vi "Options Changed.vi"(9 "error in (no error)":errorcluster, 13 "Setting ID":T1=enum."P 2") -> (8 "Settings Updated":bool, 10 "error out":errorcluster)   [LabVIEW 2011]
uses:
  Options PageID.ctl
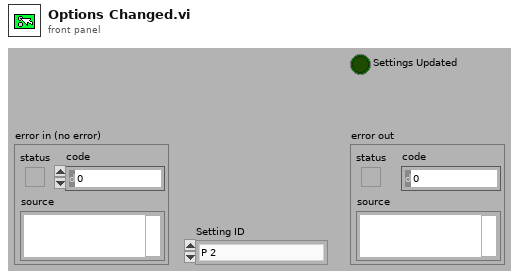
[diagram p1: front panel]
types:
  T1 = typedef "Options PageID.ctl" = enum16{"P 1 (App)", "P 2", "P 3", "P 4", "P 5", "P 6 (Err)", "P 7 (Expert)", "C 1", "C 2"}
  T2 = enum16{"Set Changed", "Changed?", "Init(numb in Prev..)"}
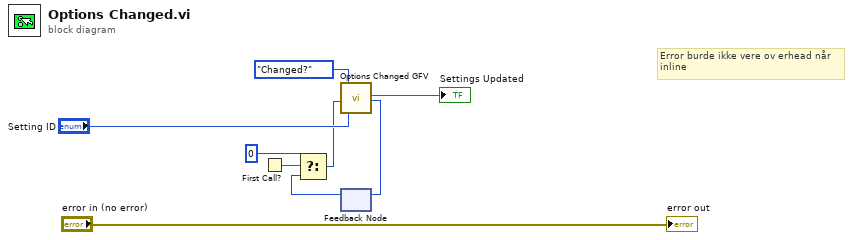
[diagram p0: block diagram]
diagram:
  # "Error burde ikke vere ov erhead når\ninline"
  n1 = First Call?() -> (First Call?: T/F=w6:bool)
  n2 = feedback #1() -> (w4:i32)  [unwired: 1 in]
  n3 = Select(t=0, s=w6, f=w4) -> (s? t:f=w2:i32)
  n4 = call "Options Changed GFV .vi"("Previous Change No"=w2, "Action(Changed?)"=T2."Changed?", "Setting ID"="Setting ID") -> ("Settings Updated"=→"Settings Updated":bool, "Change No"=w5:i32)  [unwired: 15 in]
  n5 = feedback-in #1(w5) -> ()
  "error out" <- "error in (no error)"
